vi "poly_loop_timeout_bool_i.vi"(2 "timeout (2k ms)":i32=2000, 3 "i (reset @ 0)":i32) -> (7 "timeout":bool)   [LabVIEW 2015]
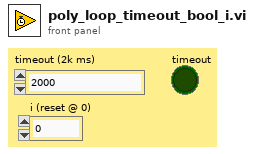
[diagram p1: front panel]
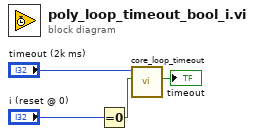
[diagram p0: block diagram]
diagram:
  n1 = Equal To 0?(x="i (reset @ 0)") -> (x = 0?=w1:bool)
  n2 = call "core_loop_timeout.vi"("i (reset @ 0)"=w1, "timeout (2k ms)"="timeout (2k ms)") -> ("timeout"=→"timeout":bool)  [unwired: 7 in, 1 out]
